vi "Filter and Data Scalingold1.vi"(0 "Offset Data":string[](array[string]), 5 "Slope Data":string[](array[string]), 7 "Filter Data":string[](array[string]), 9 "Vin":dbl[](array[numeric]), 11 "error in":errorcluster, 12 "Allow Zero?":string[](array[string])) -> (4 "Vout":string[](array[string]), 6 "Offset Data":string[](array[string]), 8 "ScaledOut":string[](array[string]), 10 "ScaledOut":dbl[](array[numeric]), 14 "Allow Zero?":string[](array[string]), 15 "error out":errorcluster)   [LabVIEW 2018]
uses:
  Counters.vi
  <vilib>/ptbypt/NI_PtbyPt.lvlib
panel:
  # "32-51= FM1 GPM Data Point 1-20"
  # "32-51= FM1 Data Point # 1-20"
  # "32-51 = FM1 K Factor 1-20"
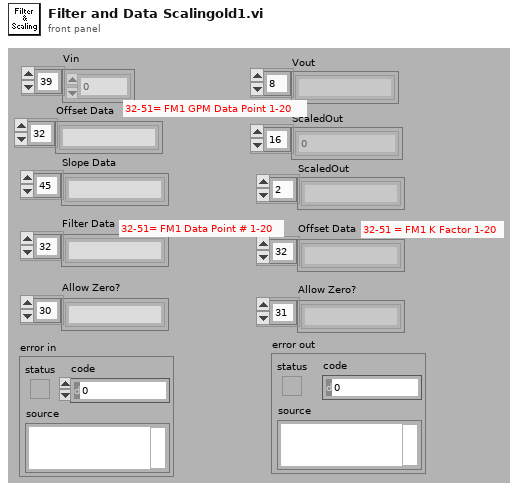
[diagram p1: front panel]
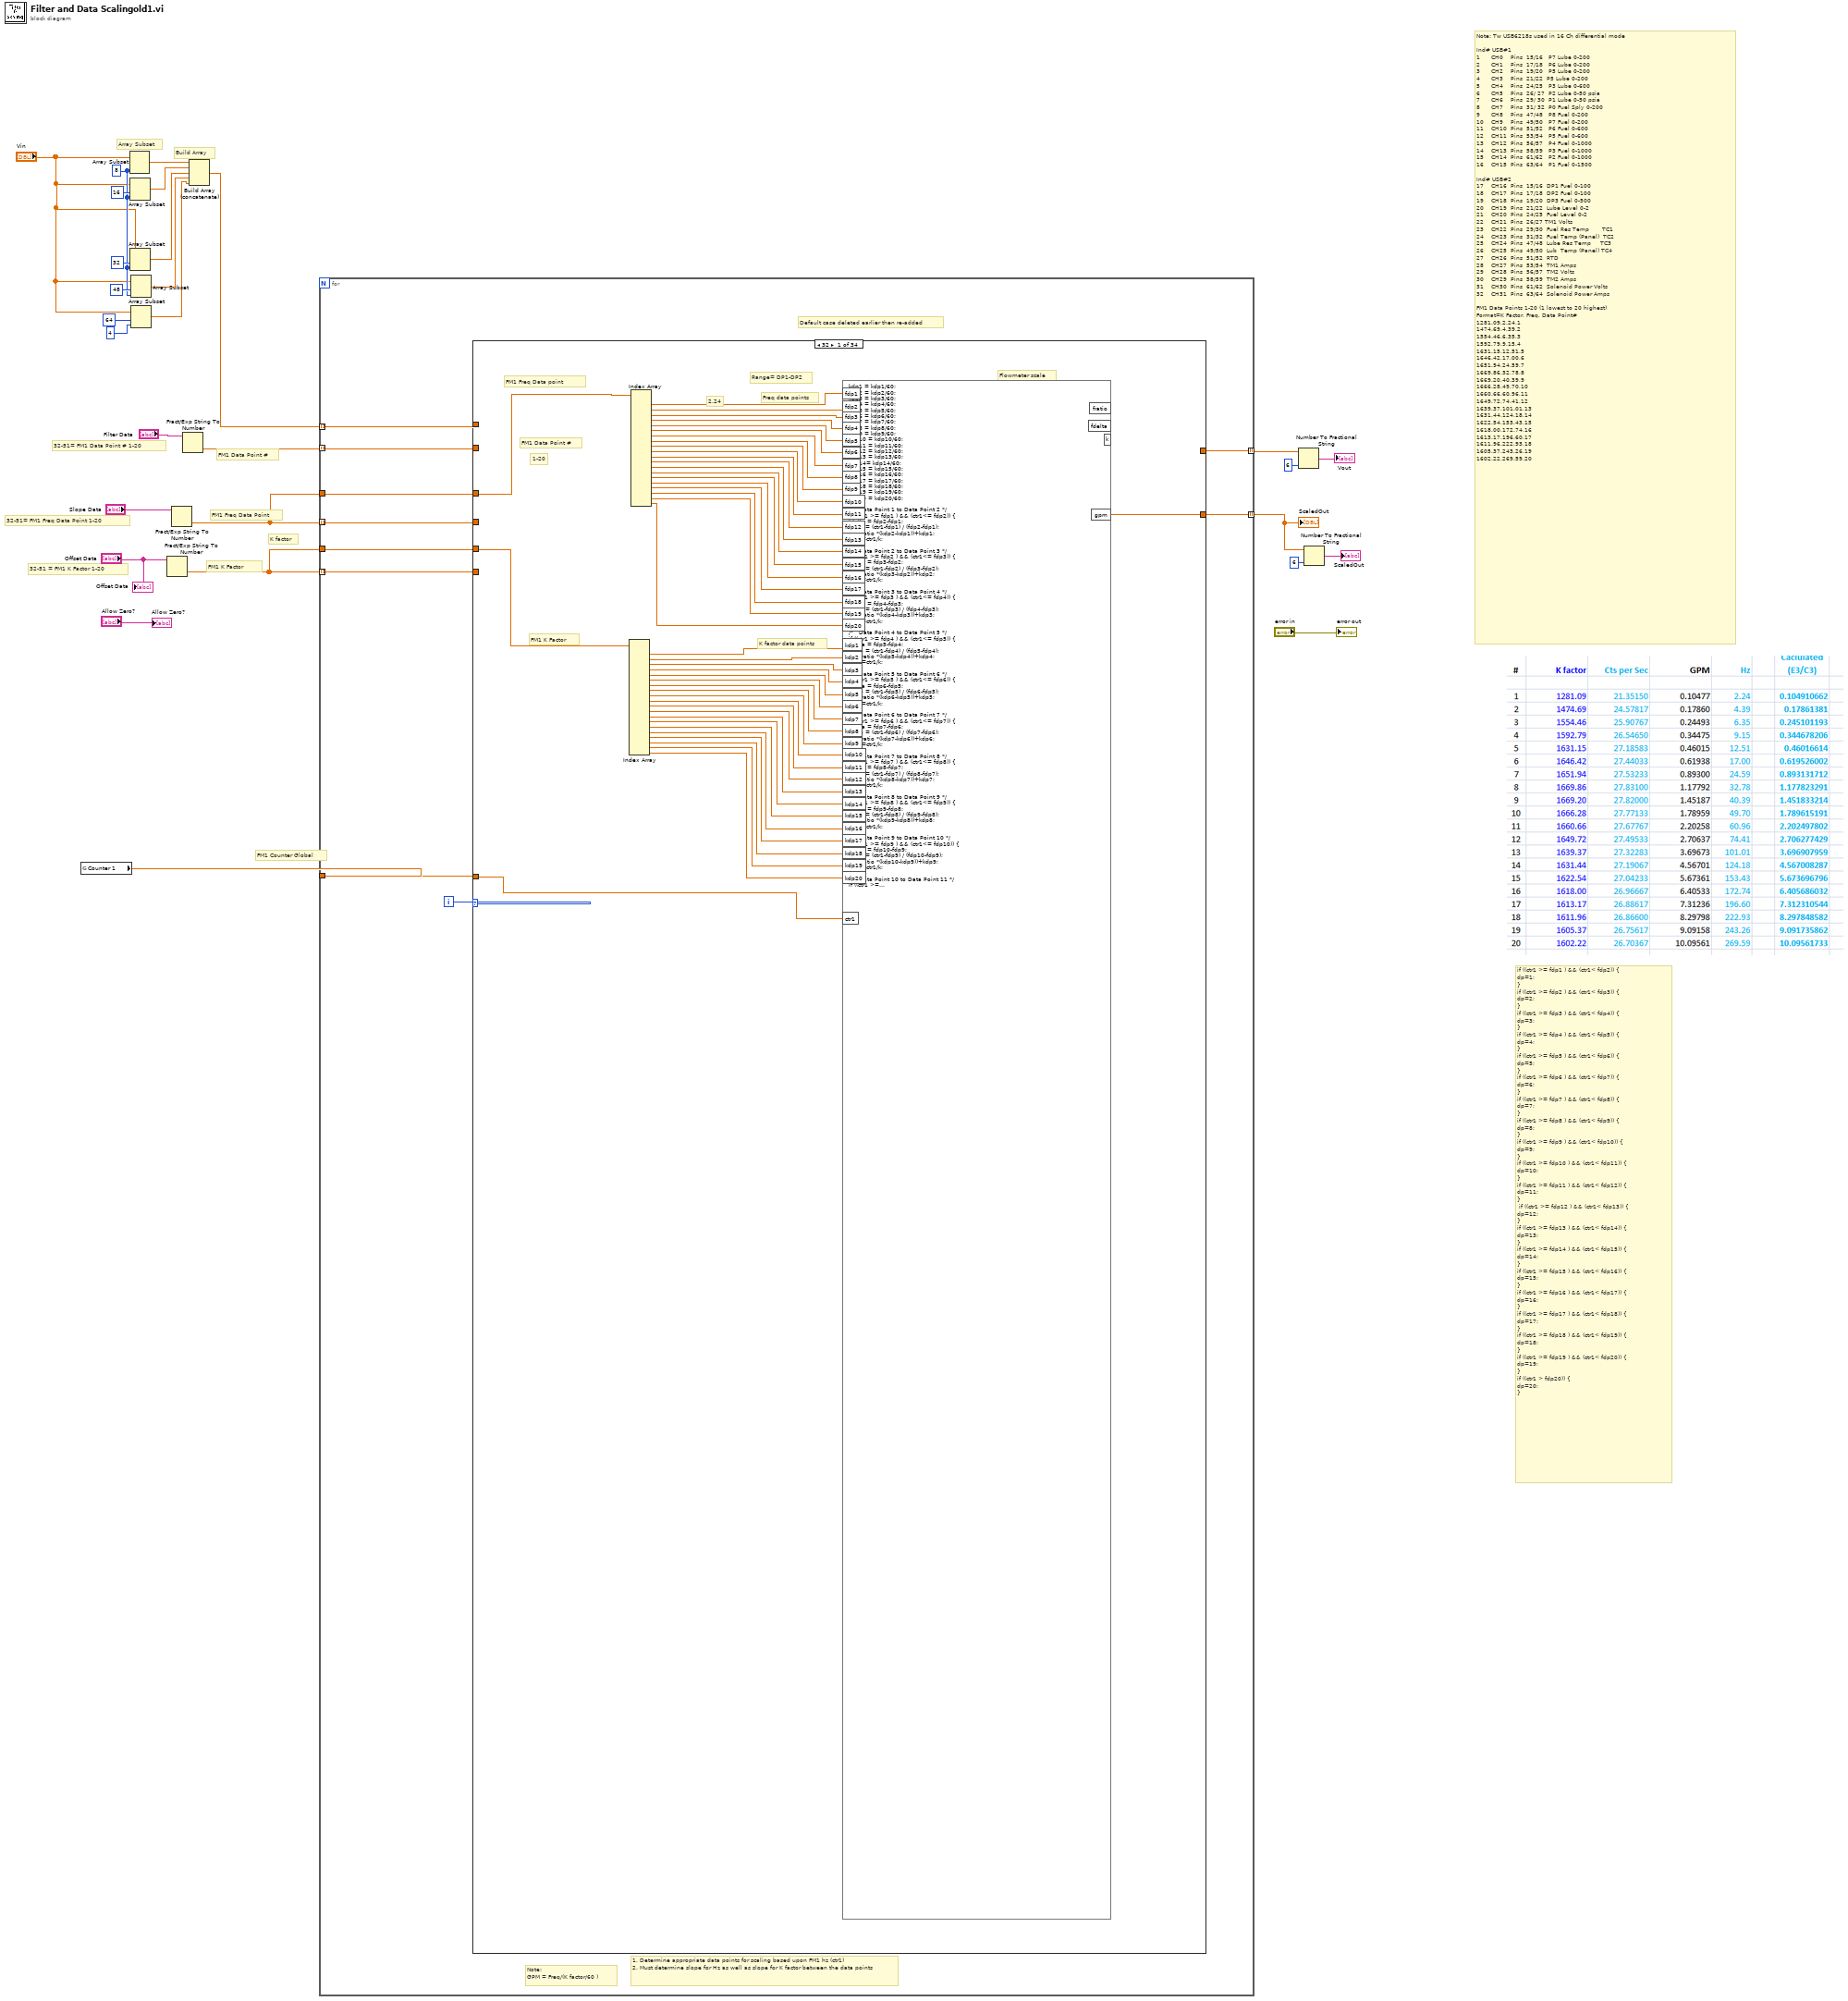
[diagram p0: block diagram]
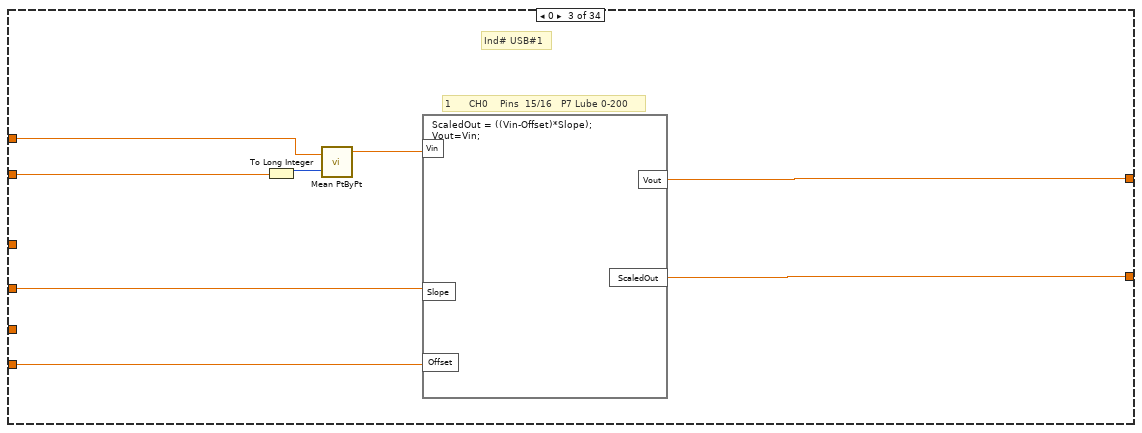
[diagram p3: hidden frame]
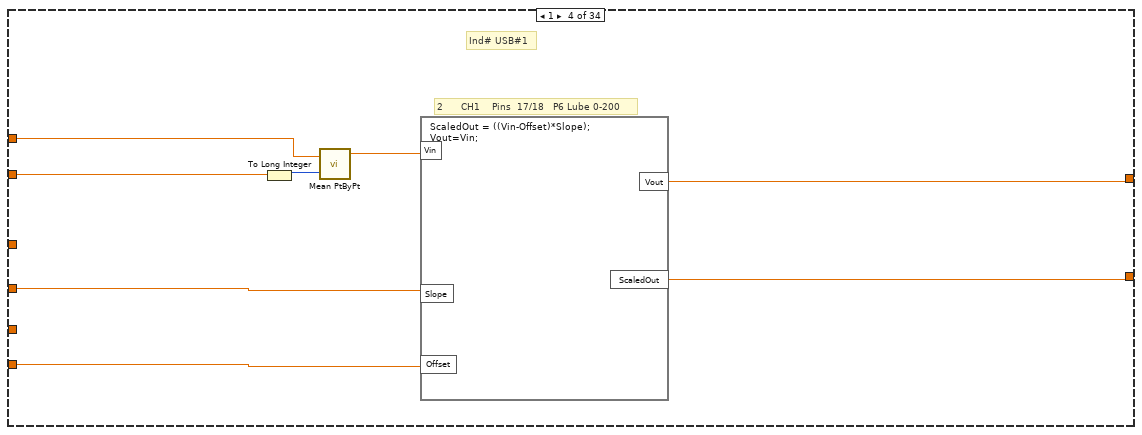
[diagram p4: hidden frame]
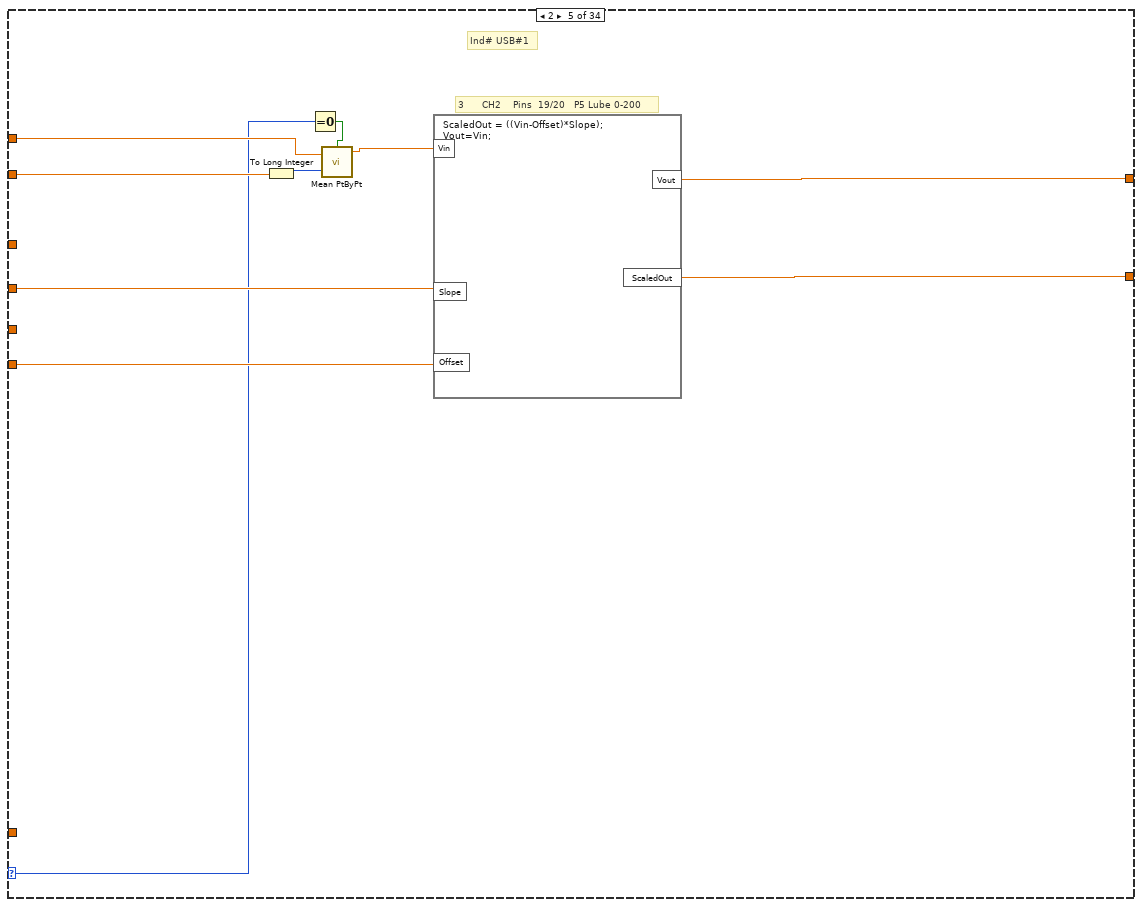
[diagram p5: hidden frame]
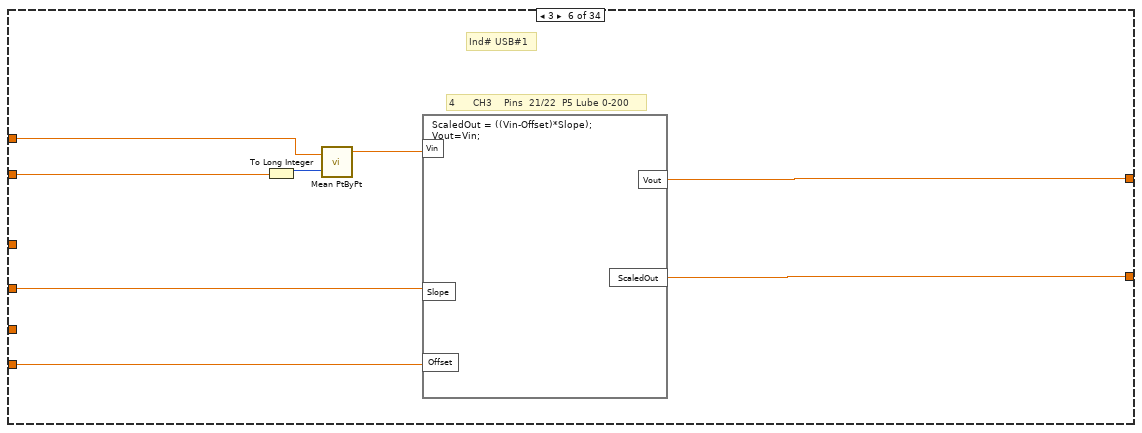
[diagram p6: hidden frame]
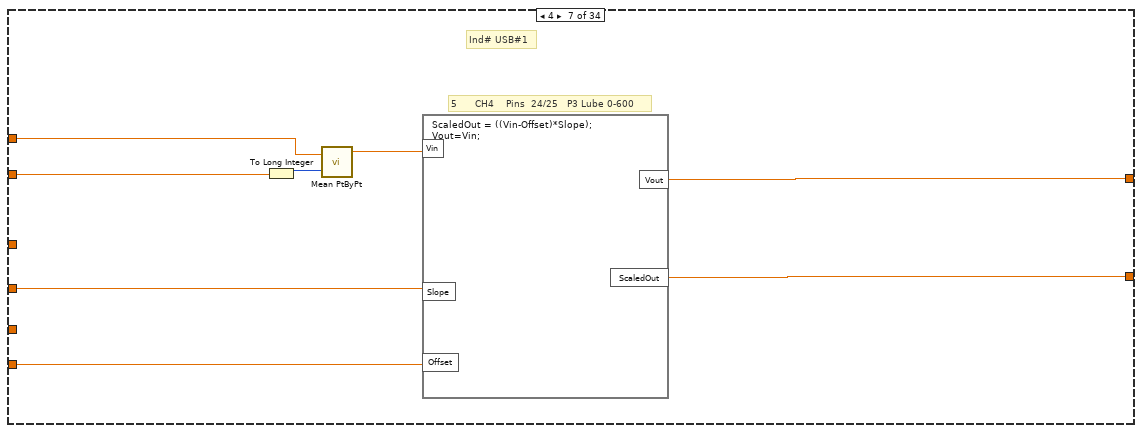
[diagram p7: hidden frame]
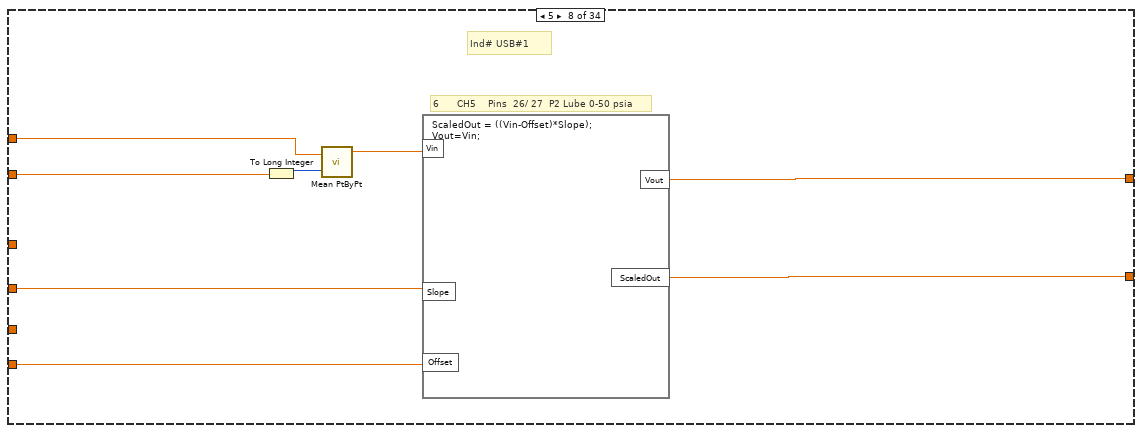
[diagram p8: hidden frame]
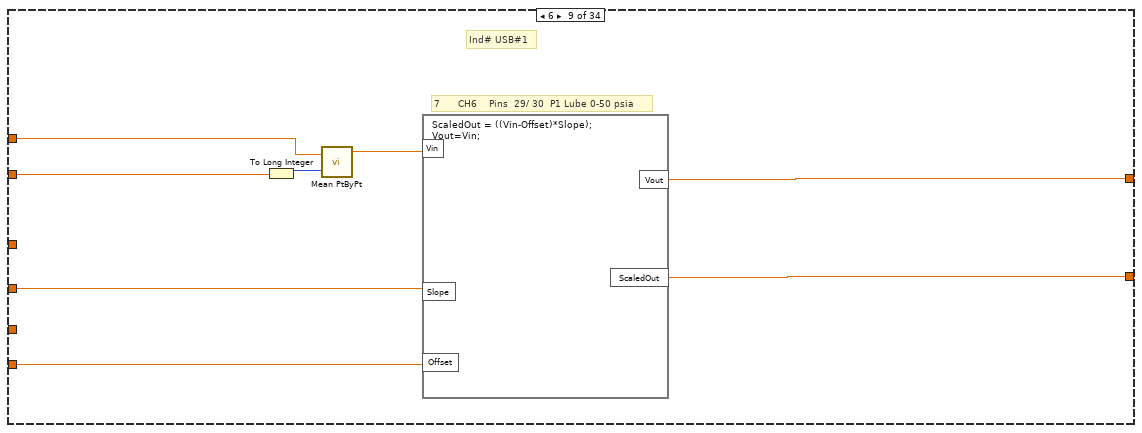
[diagram p9: hidden frame]
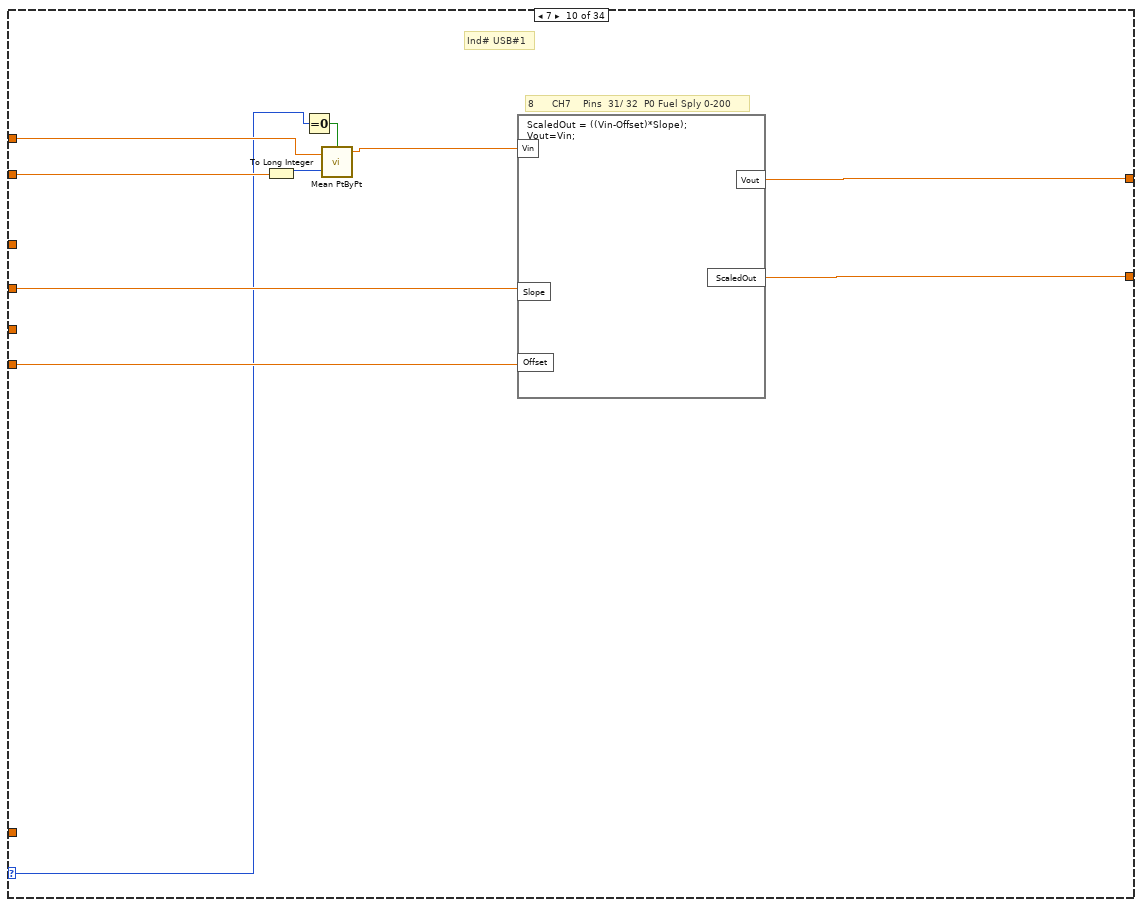
[diagram p10: hidden frame]
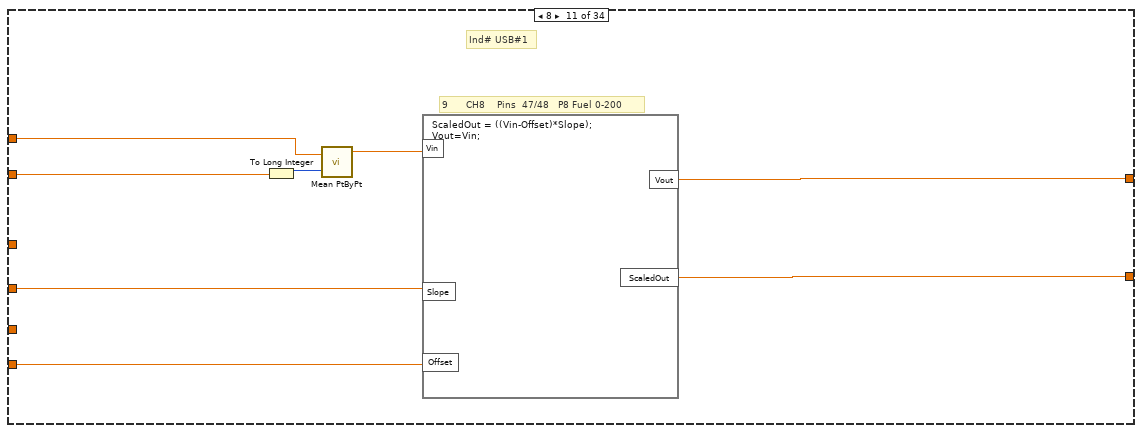
[diagram p11: hidden frame]
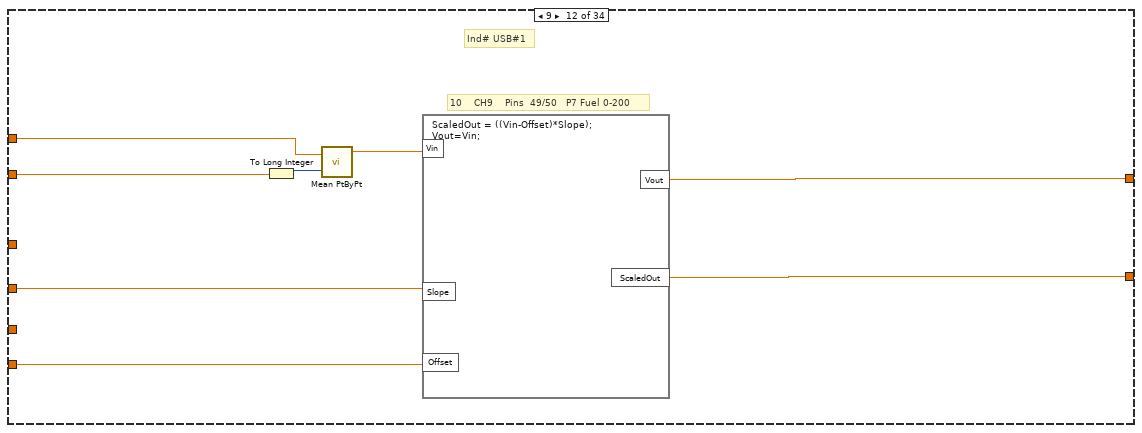
[diagram p12: hidden frame]
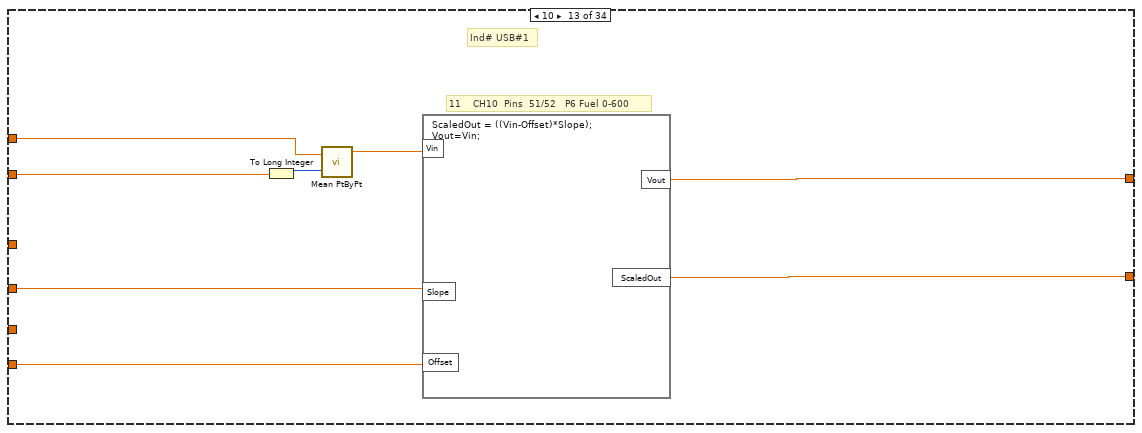
[diagram p13: hidden frame]
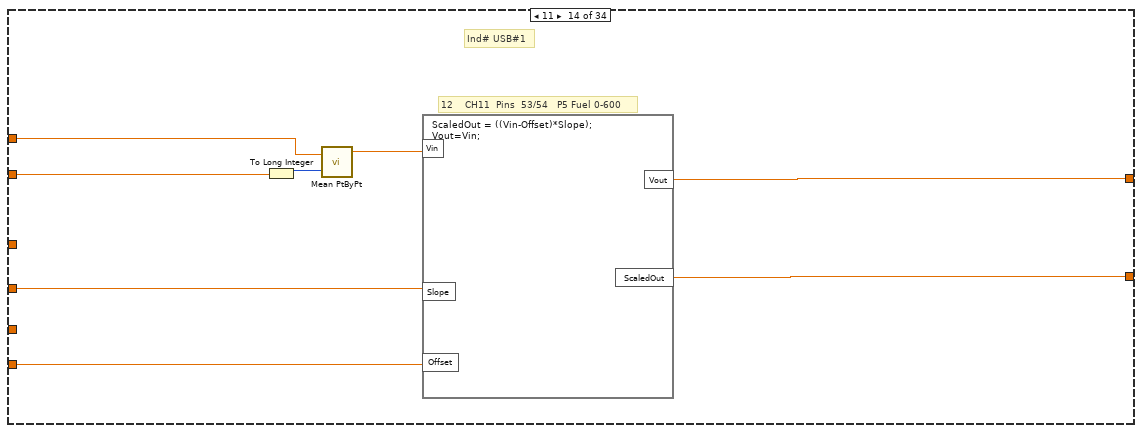
[diagram p14: hidden frame]
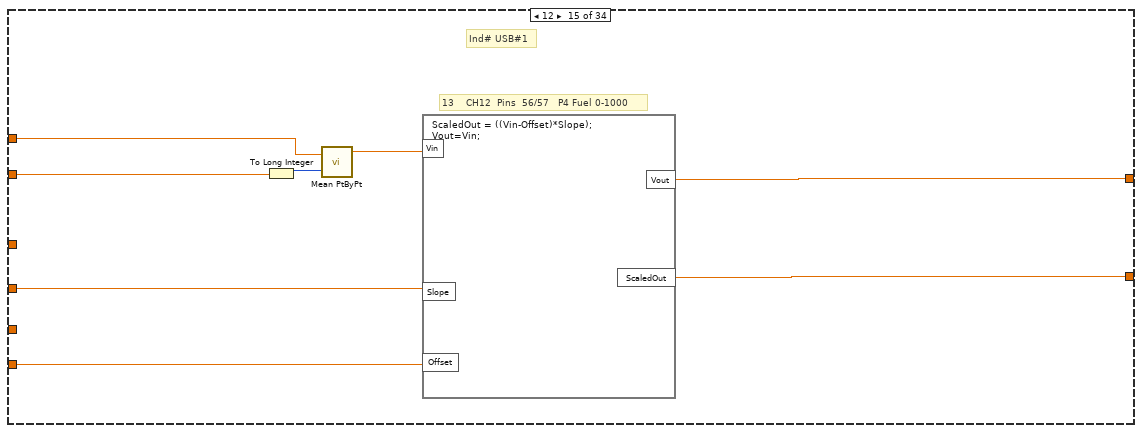
[diagram p15: hidden frame]
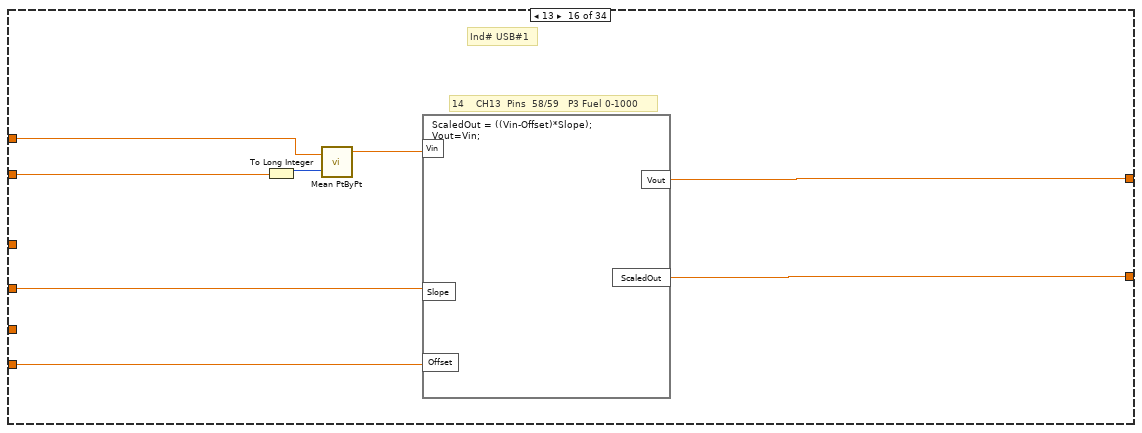
[diagram p16: hidden frame]
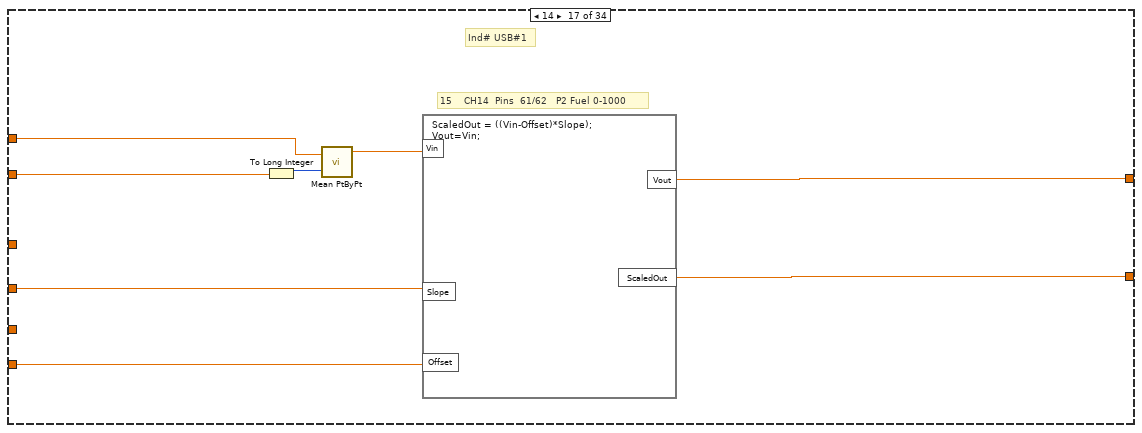
[diagram p17: hidden frame]
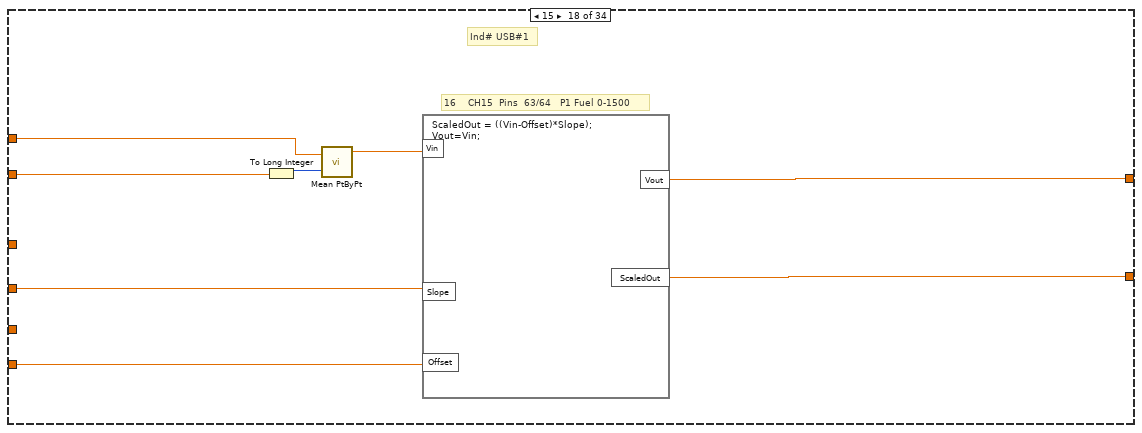
[diagram p18: hidden frame]
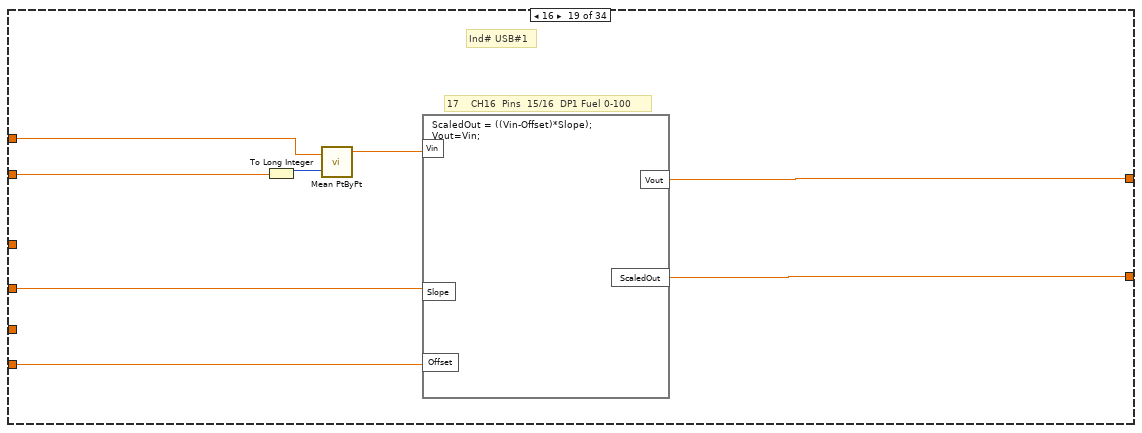
[diagram p19: hidden frame]
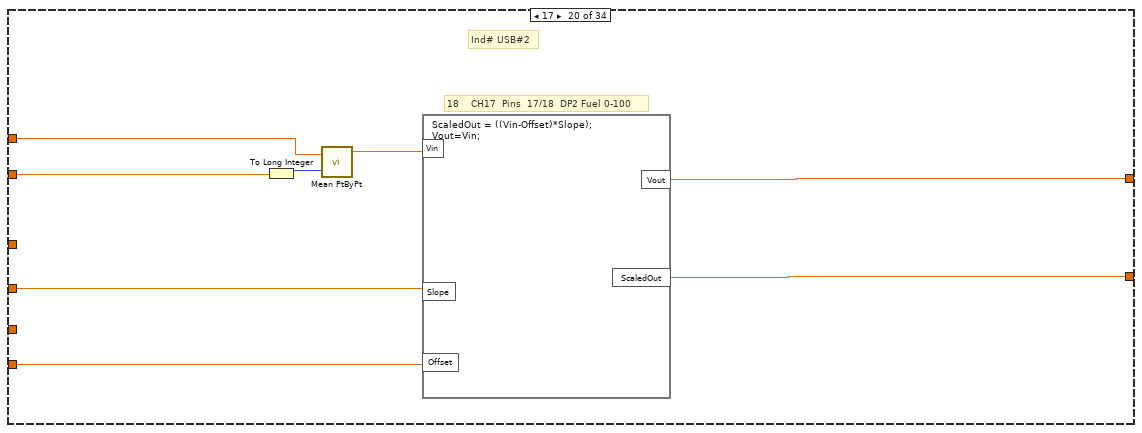
[diagram p20: hidden frame]
diagram:
  w11 = 8 ("length")
  # "if ((ctr1 >= fdp1 ) && (ctr1< fdp2)) {\ndp=1;\n}\nif ((ctr1 >= fdp2 ) && (ctr1< fdp3)) {\ndp=2;\n}\nif ((ctr1 >= fdp3 ) && (ctr1< fdp4)) {\ndp=3;\n}\nif ((ctr1 >= fdp4 ) && (ctr1< fdp5)) {\ndp=4;\n}\nif ((ctr1 >= fdp5 ) && (ctr1< fdp6)) {\ndp=5;\n}\nif ((ctr1 >= fdp6 ) && (ctr1< fdp7)) {\ndp=6;\n}\nif ((ctr1 >= fdp7 ) && (ctr1< fdp8)) {\ndp=7;\n}\nif ((ctr1 >= fdp8 ) && (ctr1< fdp9)) {\ndp=8;\n}\nif ((ctr1 >= fdp9 ) && (ctr1< fdp10)) {\ndp=9;\n}\nif ((ctr1 >= fdp10 ) && (ctr1< fdp11)) {\ndp=10;\n}\nif ((ctr1 >= fdp11 ) && (ctr1< fdp12)) {\ndp=11;\n}\n if ((ctr1 >= fdp12 ) && (ctr1< fdp13)) {\ndp=12;\n}\nif ((ctr1 >= fdp13 ) && (ctr1< fdp14)) {\ndp=13;\n}\nif ((ctr1 >= fdp14 ) && (ctr1< fdp15)) {\ndp=14;\n}\nif ((ctr1 >= fdp15 ) && (ctr1< fdp16)) {\ndp=15;\n}\nif ((ctr1 >= fdp16 ) && (ctr1< fdp17)) {\ndp=16;\n}\nif ((ctr1 >= fdp17 ) && (ctr1< fdp18)) {\ndp=17;\n}\nif ((ctr1 >= fdp18 ) && (ctr1< fdp19)) {\ndp=18;\n}\nif ((ctr1 >= fdp19 ) && (ctr1< fdp20)) {\ndp=19;\n}\nif ((ctr1 > fdp20)) {\ndp=20;\n}"
  # "Note: Tw USB6218s used in 16 Ch differential mode\n\nInd# USB#1\n1      CH0\t\t  Pins  15/16\t  P7 Lube 0-200\n2      CH1\t\t  Pins  17/18\t  P6 Lube 0-200\n3      CH2\t\t  Pins  19/20   P5 Lube 0-200\n4      CH3\t\t  Pins  21/22  P5 Lube 0-200\n5      CH4\t   Pins  24/25\t  P3 Lube 0-600\n6      CH5\t\t  Pins  26/\t27\t P2 Lube 0-50 psia\n7      CH6\t   Pins  29/\t30\t P1 Lube 0-50 psia\n8      CH7\t  \tPins  31/ 32\t P0 Fuel Sply 0-200  \n9      CH8\t  \tPins  47/48\t  P8 Fuel 0-200   \n10    CH9\t\t  Pins  49/50\t  P7 Fuel 0-200   \n11    CH10\t\tPins  51/52\t  P6 Fuel 0-600   \n12    CH11\t\tPins  53/54\t  P5 Fuel 0-600   \n13    CH12\t\tPins  56/57\t  P4 Fuel 0-1000 \n14    CH13\t\tPins  58/59\t  P3 Fuel 0-1000 \n15    CH14\t\tPins  61/62 \t P2 Fuel 0-1000  \n16    CH15\t\tPins  63/64 \t P1 Fuel 0-1500 \n\nInd# USB#2\n17    CH16\t\tPins  15/16\t DP1 Fuel 0-100 \n18    CH17\t\tPins  17/18\t DP2 Fuel 0-100\n19    CH18\t\tPins  19/20  DP3 Fuel 0-500 \n20    CH19\t Pins  21/22\t Lube Level 0-2 \n21    CH20\t\tPins  24/25\t Fuel Level 0-2 \n22    CH21\t\tPins  26/27\tTM1 Volts  \n23    CH22\t Pins  29/30  Fuel Res Temp       TC1\n24    CH23\t\tPins  31/32\t Fuel Temp (Panel)  TC2 \n25    CH24\t\tPins \t47/48\t Lube Res Temp     TC3 \n26    CH25\t\tPins  49/50\t Lub  Temp (Panel) TC4 \n27    CH26\t\tPins  51/52\t RTD \n28    CH27\t\tPins  53/54\t TM1 Amps \n29    CH28\t\tPins  56/57\t TM2 Volts\n30    CH29\t\tPins  58/59\t TM2 Amps \n31    CH30\t\tPins  61/62  Solenoid Power Volts \n32    CH31\t\tPins  63/64  Solenoid Power Amps\n\nFM1 Data Points 1-20 (1 lowest to 20 highest)\nFormat=K Factor, Freq, Data Point#\n1281.09,2.24,1\n1474.69,4.39,2\n1554.46,6.35,3\n1592.79,9.15,4\n1631.15,12.51,5\n1646.42,17.00,6\n1651.94,24.59,7\n1669.86,32.78,8\n1669.20,40.39,9\n1666.28,49.70,10\n1660.66,60.96,11\n1649.72,74.41,12\n1639.37,101.01,13\n1631.44,124.18,14\n1622.54,153.43,15\n1618.00,172.74,16\n1613.17,196.60,17\n1611.96,222.93,18\n1605.37,243.26,19\n1602.22,269.59,20"
  # "K factor"
  # "FM1 Freq Data Point"
  # "FM1 Counter Global"
  # "FM1 Data Point #"
  # "FM1 K Factor"
  # "32-51 = FM1 K Factor 1-20"
  # "32-51= FM1 Data Point # 1-20"
  # "32-51= FM1 Freq Data Point 1-20"
  # "Array Subset"
  # "Build Array"
  n1 = global read "Counters.vi" "Counter 1"() -> (w2:dbl)
  n2 = Array Subset(array="Vin", length=w11) -> (w16:dbl[])  [unwired: 1 in]
  n3 = Array Subset(array="Vin", index=16, length=w11) -> (w15:dbl[])
  n4 = Array Subset(array="Vin", index=32, length=w11) -> (w13:dbl[])
  n5 = Array Subset(array="Vin", index=48, length=w11) -> (w14:dbl[])
  n6 = Array Subset(array="Vin", index=64, length=4 ("index")) -> (w6:dbl[])
  n7 = Fract/Exp String To Number(string="Offset Data") -> (number=w3:dbl[])  [unwired: 4 out]
  n8 = Fract/Exp String To Number(string="Slope Data") -> (number=w4:dbl[])  [unwired: 4 out]
  n9 = Fract/Exp String To Number(string="Filter Data") -> (number=w1:dbl[])  [unwired: 4 out]
  n10 = Build Array (concatenate)(w16, w15, w13, w14, w6) -> (w5:dbl[])
  n11 = for {
    tunnel: w4 -> [w37] mode=indexing
    tunnel: w3 -> [w32] mode=indexing
    tunnel: w1 -> [w38] mode=indexing
    tunnel: [w35] -> w10 mode=indexing
    tunnel: [w36] -> w19 mode=indexing
    tunnel: w5 -> [w33] mode=indexing
    tunnel: w4 -> [w31]
    tunnel: w3 -> [w30]
    tunnel: w2 -> [w29]
    i -> [w34]
    # "Note:\nGPM = Freq/(K factor/60 )"
    # "1. Determine appropriate data points for scaling based upon FM1 hz (ctr1)\n2. Must determine slope for Hz as well as slope for K factor between the data points"
    # "Default case deleted earlier then re-added"
    n12 = case shown="32" w34 {
      selector: w34 -> [_ _ _ _ w102 _ _ _ _ w144 _ _ _ _ _ _ _ _ _ _ _ _ _ _ _ _ _ _ _ _ _ _ _ _]
      tunnel: w33 -> [_ _ w87 w93 w107 w113 w121 w129 w137 w149 w155 w163 w171 w179 w187 w195 w203 w211 w219 w227 w235 w243 w251 w259 w267 w275 w283 w291 w299 w307 w315 w323 w331 w339]
      tunnel: w38 -> [_ _ w88 w94 w108 w114 w122 w130 w138 w150 w156 w164 w172 w180 w188 w196 w204 w212 w220 w228 w236 w244 w252 w260 w268 w276 w284 w292 w300 w308 w316 w324 w332 w340]
      tunnel: w37 -> [_ _ w86 w96 w106 w112 w120 w128 w136 w148 w154 w162 w170 w178 w186 w194 w202 w210 w218 w226 w234 w242 w250 w258 w266 w274 w282 w290 w298 w306 w314 w322 w330 w338]
      tunnel: w32 -> [_ _ w85 w95 w105 w111 w119 w127 w135 w147 w153 w161 w169 w177 w185 w193 w201 w209 w217 w225 w233 w241 w249 w257 w265 w273 w281 w289 w297 w305 w313 w321 w329 w337]
      tunnel: [_ _ w83 w92 w103 w109 w117 w125 w133 w145 w151 w159 w167 w175 w183 w191 w199 w207 w215 w223 w231 w239 w247 w255 w263 w271 w279 w287 w295 w303 w311 w319 w327 w335] -> w36
      tunnel: [w79 _ w84 w91 w104 w110 w118 w126 w134 w146 w152 w160 w168 w176 w184 w192 w200 w208 w216 w224 w232 w240 w248 w256 w264 w272 w280 w288 w296 w304 w312 w320 w328 w336] -> w35
      tunnel: w31 -> [w81 _ _ _ _ _ _ _ _ _ _ _ _ _ _ _ _ _ _ _ _ _ _ _ _ _ _ _ _ _ _ _ _ _]
      tunnel: w30 -> [w80 _ _ _ _ _ _ _ _ _ _ _ _ _ _ _ _ _ _ _ _ _ _ _ _ _ _ _ _ _ _ _ _ _]
      tunnel: w29 -> [w82 _ _ _ _ _ _ _ _ _ _ _ _ _ _ _ _ _ _ _ _ _ _ _ _ _ _ _ _ _ _ _ _ _]
      frame 32 {
        # "2.24"
        # "Range= DP1-DP2"
        # "K factor data points"
        # "Freq data points"
        # "Flowmeter scale"
        # "1-20"
        # "FM1 Data Point #"
        # "FM1 K Factor"
        # "FM1 Freq Data point"
        n13 = Index Array(array=w80) -> (element #1=w58:dbl, element #2=w57:dbl, element #3=w56:dbl, element #4=w55:dbl, element #5=w54:dbl, element #6=w53:dbl, element #7=w52:dbl, element #8=w51:dbl, element #9=w50:dbl, element #10=w49:dbl, element #11=w48:dbl, element #12=w47:dbl, element #13=w46:dbl, element #14=w45:dbl, element #15=w44:dbl, element #16=w43:dbl, element #17=w42:dbl, element #18=w41:dbl, element #19=w40:dbl, element #20=w39:dbl)  [unwired: 20 in]
        n14 = Index Array(array=w81) -> (element #1=w78:dbl, element #2=w77:dbl, element #3=w76:dbl, element #4=w75:dbl, element #5=w74:dbl, element #6=w73:dbl, element #7=w72:dbl, element #8=w71:dbl, element #9=w70:dbl, element #10=w69:dbl, element #11=w68:dbl, element #12=w67:dbl, element #13=w66:dbl, element #14=w65:dbl, element #15=w64:dbl, element #16=w63:dbl, element #17=w62:dbl, element #18=w61:dbl, element #19=w60:dbl, element #20=w59:dbl)  [unwired: 20 in]
        n15 = formula code="kdp1 = kdp1/60;\nkdp2 = kdp2/60;\nkdp3 = kdp3/60;\nkdp4 = kdp4/60;\nkdp5 = kdp5/60;\nkdp6 = kdp6/60;\nkdp7 = kdp7/60;\nkdp8 = kdp8/60;\nkdp9 = kdp9/60;\nkdp10 = kdp10/60;\nkdp11 = kdp11/60;\nkdp12 = kdp12/60;\nkdp13 = kdp13/60;\nkdp14= kdp14/60;\nkdp15 = kdp15/60;\nkdp16 = kdp16/60;\nkdp17 = kdp17/60;\nkdp18 = kdp18/60;\nkdp19 = kdp19/60;\nkdp20 = kdp20/60;\n\n/*   Data Point 1 to Data Point 2 */\nif ((ctr1 >= fdp1 ) && (ctr1<= fdp2)) {\nfdelta = fdp2-fdp1;\nfratio = (ctr1-fdp1) / (fdp2-fdp1);\nk =(fratio *(kdp2-kdp1))+kdp1;\ngpm=ctr1/k;\n}\n/*   Data Point 2 to Data Point 3 */\nif ((ctr1 >= fdp2 ) && (ctr1<= fdp3)) {\nfdelta = fdp3-fdp2;\nfratio = (ctr1-fdp2) / (fdp3-fdp2);\nk =(fratio *(kdp3-kdp2))+kdp2;\ngpm=ctr1/k;\n}\n/*   Data Point 3 to Data Point 4 */\nif ((ctr1 >= fdp3 ) && (ctr1<= fdp4)) {\nfdelta = fdp4-fdp3;\nfratio = (ctr1-fdp3) / (fdp4-fdp3);\nk =(fratio *(kdp4-kdp3))+kdp3;\ngpm=ctr1/k;\n}\n/*   Data Point 4 to Data Point 5 */\nif ((ctr1 >= fdp4 ) && (ctr1<= fdp5)) {\nfdelta = fdp5-fdp4;\nfratio = (ctr1-fdp4) / (fdp5-fdp4);\nk =(fratio *(kdp5-kdp4))+kdp4;\ngpm=ctr1/k;\n}\n/*   Data Point 5 to Data Point 6 */\nif ((ctr1 >= fdp5 ) && (ctr1<= fdp6)) {\nfdelta = fdp6-fdp5;\nfratio = (ctr1-fdp5) / (fdp6-fdp5);\nk =(fratio *(kdp6-kdp5))+kdp5;\ngpm=ctr1/k;\n}\n/*   Data Point 6 to Data Point 7 */\nif ((ctr1 >= fdp6 ) && (ctr1<= fdp7)) {\nfdelta = fdp7-fdp6;\nfratio = (ctr1-fdp6) / (fdp7-fdp6);\nk =(fratio *(kdp7-kdp6))+kdp6;\ngpm=ctr1/k;\n}\n/*   Data Point 7 to Data Point 8 */\nif ((ctr1 >= fdp7 ) && (ctr1<= fdp8)) {\nfdelta = fdp8-fdp7;\nfratio = (ctr1-fdp7) / (fdp8-fdp7);\nk =(fratio *(kdp8-kdp7))+kdp7;\ngpm=ctr1/k;\n}\n/*   Data Point 8 to Data Point 9 */\nif ((ctr1 >= fdp8 ) && (ctr1<= fdp9)) {\nfdelta = fdp9-fdp8;\nfratio = (ctr1-fdp8) / (fdp9-fdp8);\nk =(fratio *(kdp9-kdp8))+kdp8;\ngpm=ctr1/k;\n}\n/*   Data Point 9 to Data Point 10 */\nif ((ctr1 >= fdp9 ) && (ctr1<= fdp10)) {\nfdelta = fdp10-fdp9;\nfratio = (ctr1-fdp9) / (fdp10-fdp9);\nk =(fratio *(kdp10-kdp9))+kdp9;\ngpm=ctr1/k;\n}\n/*   Data Point 10 to Data Point 11 */\nif ((ctr1 >= fdp10 ) && (ctr1<= fdp11)) {\nfdelta = fdp11-fdp10;\nfratio = (ctr1-fdp10) / (fdp11-fdp10);\nk =(fratio *(kdp11-kdp10))+kdp10;\ngpm=ctr1/k;\n}\n/*   Data Point 11 to Data Point 12 */\nif ((ctr1 >= fdp11 ) && (ctr1<= fdp12)) {\nfdelta = fdp12-fdp11;\nfratio = (ctr1-fdp11) / (fdp12-fdp11);\nk =(fratio *(kdp12-kdp11))+kdp11;\ngpm=ctr1/k;\n}\n/*   Data Point 12 to Data Point 13 */\nif ((ctr1 >= fdp12) && (ctr1<= fdp13)) {\nfdelta = fdp13-fdp12;\nfratio = (ctr1-fdp12) / (fdp13-fdp12);\nk =(fratio *(kdp13-kdp12))+kdp12;\ngpm=ctr1/k;\n}\n/*   Data Point 13 to Data Point 14 */\nif ((ctr1 >= fdp13 ) && (ctr1<= fdp14)) {\nfdelta = fdp14-fdp13;\nfratio = (ctr1-fdp13) / (fdp14-fdp13);\nk =(fratio *(kdp14-kdp13))+kdp13;\ngpm=ctr1/k;\n}\nif ((ctr1 >= fdp14 ) && (ctr1<= fdp15)) {\nfdelta = fdp15-fdp14;\nfratio = (ctr1-fdp14) / (fdp15-fdp14);\nk =(fratio *(kdp15-kdp14))+kdp14;\ngpm=ctr1/k;\n}\n/*   Data Point 15 to Data Point 16 */\nif ((ctr1 >= fdp15 ) && (ctr1<= fdp16)) {\nfdelta = fdp16-fdp15;\nfratio = (ctr1-fdp15) / (fdp16-fdp15);\nk =(fratio *(kdp16-kdp15))+kdp15;\ngpm=ctr1/k;\n}\n/*   Data Point 16 to Data Point 17 */\nif ((ctr1 >= fdp16 ) && (ctr1<= fdp17)) {\nfdelta = fdp17-fdp16;\nfratio = (ctr1-fdp16) / (fdp17-fdp16);\nk =(fratio *(kdp17-kdp16))+kdp16;\ngpm=ctr1/k;\n}\n/*   Data Point 17 to Data Point 18 */\nif ((ctr1 >= fdp17 ) && (ctr1<= fdp18)) {\nfdelta = fdp18-fdp17;\nfratio = (ctr1-fdp17) / (fdp18-fdp17);\nk =(fratio *(kdp18-kdp17))+kdp17;\ngpm=ctr1/k;\n}\n/*   Data Point 18 to Data Point 19 */\nif ((ctr1 >= fdp18 ) && (ctr1<= fdp19)) {\nfdelta = fdp19-fdp18;\nfratio = (ctr1-fdp18) / (fdp19-fdp18);\nk =(fratio *(kdp19-kdp18))+kdp18;\ngpm=ctr1/k;\n}\n/*   Data Point 19 to Data Point 20 */\nif ((ctr1 >= fdp19 ) && (ctr1<= fdp20)) {\nfdelta = fdp20-fdp19;\nfratio = (ctr1-fdp19) / (fdp20-fdp19);\nk =(fratio *(kdp20-kdp19))+kdp19;\ngpm=ctr1/k;\n}\n\nif (ctr1 < fdp1) {  /*  Handles frequency < lowest on table */ \ngpm =0;\n}"("fdp1"=w78, "fdp2"=w77, "kdp1"=w58, "ctr1"=w82, "kdp2"=w57, "fdp3"=w76, "fdp4"=w75, "fdp5"=w74, "fdp6"=w73, "fdp7"=w72, "fdp8"=w71, "fdp9"=w70, "fdp10"=w69, "fdp11"=w68, "fdp12"=w67, "fdp13"=w66, "fdp14"=w65, "fdp15"=w64, "fdp16"=w63, "fdp17"=w62, "fdp18"=w61, "fdp19"=w60, "fdp20"=w59, "kdp3"=w56, "kdp4"=w55, "kdp5"=w54, "kdp6"=w53, "kdp7"=w52, "kdp8"=w51, "kdp9"=w50, "kdp10"=w49, "kdp11"=w48, "kdp12"=w47, "kdp13"=w46, "kdp14"=w45, "kdp15"=w44, "kdp16"=w43, "kdp17"=w42, "kdp18"=w41, "kdp19"=w40, "kdp20"=w39) -> ("gpm"=w79:dbl)  [unwired: 3 out]
      }
      frame 33, Default {
      }
      frame 0 {
        # "Ind# USB#1"
        # "1      CH0\t\t  Pins  15/16\t  P7 Lube 0-200"
        n16 = To Long Integer(number=w88) -> (32bit integer=w90:i32)
        n17 = call <vilib>:"Mean PtByPt.vi"("x"=w87, "sample length"=w90) -> ("mean"=w89:dbl)  [unwired: 1 in, 2 out]
        n18 = formula code="ScaledOut = ((Vin-Offset)*Slope);\nVout=Vin;"("Vin"=w89, "Slope"=w86, "Offset"=w85) -> ("ScaledOut"=w84:dbl, "Vout"=w83:dbl)
      }
      frame 1 {
        # "Ind# USB#1"
        # "2      CH1\t\t  Pins  17/18\t  P6 Lube 0-200"
        n19 = To Long Integer(number=w94) -> (32bit integer=w98:i32)
        n20 = call <vilib>:"Mean PtByPt.vi"("x"=w93, "sample length"=w98) -> ("mean"=w97:dbl)  [unwired: 1 in, 2 out]
        n21 = formula code="ScaledOut = ((Vin-Offset)*Slope);\nVout=Vin;"("Vin"=w97, "Slope"=w96, "Offset"=w95) -> ("ScaledOut"=w91:dbl, "Vout"=w92:dbl)
      }
      frame 2 {
        # "Ind# USB#1"
        # "3      CH2\t\t  Pins  19/20   P5 Lube 0-200"
        n22 = To Long Integer(number=w108) -> (32bit integer=w101:i32)
        n23 = Equal To 0?(x=w102) -> (x = 0?=w100:bool)
        n24 = call <vilib>:"Mean PtByPt.vi"("x"=w107, "sample length"=w101, "initialize"=w100) -> ("mean"=w99:dbl)  [unwired: 2 out]
        n25 = formula code="ScaledOut = ((Vin-Offset)*Slope);\nVout=Vin;"("Vin"=w99, "Slope"=w106, "Offset"=w105) -> ("ScaledOut"=w104:dbl, "Vout"=w103:dbl)
      }
      frame 3 {
        # "Ind# USB#1"
        # "4      CH3\t\t  Pins  21/22  P5 Lube 0-200"
        n26 = To Long Integer(number=w114) -> (32bit integer=w116:i32)
        n27 = call <vilib>:"Mean PtByPt.vi"("x"=w113, "sample length"=w116) -> ("mean"=w115:dbl)  [unwired: 1 in, 2 out]
        n28 = formula code="ScaledOut = ((Vin-Offset)*Slope);\nVout=Vin;"("Vin"=w115, "Slope"=w112, "Offset"=w111) -> ("ScaledOut"=w110:dbl, "Vout"=w109:dbl)
      }
      frame 4 {
        # "Ind# USB#1"
        # "5      CH4\t   Pins  24/25\t  P3 Lube 0-600"
        n29 = To Long Integer(number=w122) -> (32bit integer=w124:i32)
        n30 = call <vilib>:"Mean PtByPt.vi"("x"=w121, "sample length"=w124) -> ("mean"=w123:dbl)  [unwired: 1 in, 2 out]
        n31 = formula code="ScaledOut = ((Vin-Offset)*Slope);\nVout=Vin;"("Vin"=w123, "Slope"=w120, "Offset"=w119) -> ("ScaledOut"=w118:dbl, "Vout"=w117:dbl)
      }
      frame 5 {
        # "6      CH5\t\t  Pins  26/\t27\t P2 Lube 0-50 psia"
        # "Ind# USB#1"
        n32 = To Long Integer(number=w130) -> (32bit integer=w132:i32)
        n33 = call <vilib>:"Mean PtByPt.vi"("x"=w129, "sample length"=w132) -> ("mean"=w131:dbl)  [unwired: 1 in, 2 out]
        n34 = formula code="ScaledOut = ((Vin-Offset)*Slope);\nVout=Vin;"("Vin"=w131, "Slope"=w128, "Offset"=w127) -> ("ScaledOut"=w126:dbl, "Vout"=w125:dbl)
      }
      frame 6 {
        # "7      CH6\t   Pins  29/\t30\t P1 Lube 0-50 psia"
        # "Ind# USB#1"
        n35 = To Long Integer(number=w138) -> (32bit integer=w140:i32)
        n36 = call <vilib>:"Mean PtByPt.vi"("x"=w137, "sample length"=w140) -> ("mean"=w139:dbl)  [unwired: 1 in, 2 out]
        n37 = formula code="ScaledOut = ((Vin-Offset)*Slope);\nVout=Vin;"("Vin"=w139, "Slope"=w136, "Offset"=w135) -> ("ScaledOut"=w134:dbl, "Vout"=w133:dbl)
      }
      frame 7 {
        # "8      CH7\t  \tPins  31/ 32\t P0 Fuel Sply 0-200"
        # "Ind# USB#1"
        n38 = To Long Integer(number=w150) -> (32bit integer=w142:i32)
        n39 = Equal To 0?(x=w144) -> (x = 0?=w143:bool)
        n40 = call <vilib>:"Mean PtByPt.vi"("x"=w149, "sample length"=w142, "initialize"=w143) -> ("mean"=w141:dbl)  [unwired: 2 out]
        n41 = formula code="ScaledOut = ((Vin-Offset)*Slope);\nVout=Vin;"("Vin"=w141, "Slope"=w148, "Offset"=w147) -> ("ScaledOut"=w146:dbl, "Vout"=w145:dbl)
      }
      frame 8 {
        # "9      CH8\t  \tPins  47/48\t  P8 Fuel 0-200"
        # "Ind# USB#1"
        n42 = To Long Integer(number=w156) -> (32bit integer=w158:i32)
        n43 = call <vilib>:"Mean PtByPt.vi"("x"=w155, "sample length"=w158) -> ("mean"=w157:dbl)  [unwired: 1 in, 2 out]
        n44 = formula code="ScaledOut = ((Vin-Offset)*Slope);\nVout=Vin;"("Vin"=w157, "Slope"=w154, "Offset"=w153) -> ("ScaledOut"=w152:dbl, "Vout"=w151:dbl)
      }
      frame 9 {
        # "10    CH9\t\t  Pins  49/50\t  P7 Fuel 0-200"
        # "Ind# USB#1"
        n45 = To Long Integer(number=w164) -> (32bit integer=w166:i32)
        n46 = call <vilib>:"Mean PtByPt.vi"("x"=w163, "sample length"=w166) -> ("mean"=w165:dbl)  [unwired: 1 in, 2 out]
        n47 = formula code="ScaledOut = ((Vin-Offset)*Slope);\nVout=Vin;"("Vin"=w165, "Slope"=w162, "Offset"=w161) -> ("ScaledOut"=w160:dbl, "Vout"=w159:dbl)
      }
      frame 10 {
        # "11    CH10\t\tPins  51/52\t  P6 Fuel 0-600"
        # "Ind# USB#1"
        n48 = To Long Integer(number=w172) -> (32bit integer=w174:i32)
        n49 = call <vilib>:"Mean PtByPt.vi"("x"=w171, "sample length"=w174) -> ("mean"=w173:dbl)  [unwired: 1 in, 2 out]
        n50 = formula code="ScaledOut = ((Vin-Offset)*Slope);\nVout=Vin;"("Vin"=w173, "Slope"=w170, "Offset"=w169) -> ("ScaledOut"=w168:dbl, "Vout"=w167:dbl)
      }
      frame 11 {
        # "12    CH11\t\tPins  53/54\t  P5 Fuel 0-600"
        # "Ind# USB#1"
        n51 = To Long Integer(number=w180) -> (32bit integer=w182:i32)
        n52 = call <vilib>:"Mean PtByPt.vi"("x"=w179, "sample length"=w182) -> ("mean"=w181:dbl)  [unwired: 1 in, 2 out]
        n53 = formula code="ScaledOut = ((Vin-Offset)*Slope);\nVout=Vin;"("Vin"=w181, "Slope"=w178, "Offset"=w177) -> ("ScaledOut"=w176:dbl, "Vout"=w175:dbl)
      }
      frame 12 {
        # "13    CH12\t\tPins  56/57\t  P4 Fuel 0-1000"
        # "Ind# USB#1"
        n54 = To Long Integer(number=w188) -> (32bit integer=w190:i32)
        n55 = call <vilib>:"Mean PtByPt.vi"("x"=w187, "sample length"=w190) -> ("mean"=w189:dbl)  [unwired: 1 in, 2 out]
        n56 = formula code="ScaledOut = ((Vin-Offset)*Slope);\nVout=Vin;"("Vin"=w189, "Slope"=w186, "Offset"=w185) -> ("ScaledOut"=w184:dbl, "Vout"=w183:dbl)
      }
      frame 13 {
        # "14    CH13\t\tPins  58/59\t  P3 Fuel 0-1000"
        # "Ind# USB#1"
        n57 = To Long Integer(number=w196) -> (32bit integer=w198:i32)
        n58 = call <vilib>:"Mean PtByPt.vi"("x"=w195, "sample length"=w198) -> ("mean"=w197:dbl)  [unwired: 1 in, 2 out]
        n59 = formula code="ScaledOut = ((Vin-Offset)*Slope);\nVout=Vin;"("Vin"=w197, "Slope"=w194, "Offset"=w193) -> ("ScaledOut"=w192:dbl, "Vout"=w191:dbl)
      }
      frame 14 {
        # "15    CH14\t\tPins  61/62 \t P2 Fuel 0-1000"
        # "Ind# USB#1"
        n60 = To Long Integer(number=w204) -> (32bit integer=w206:i32)
        n61 = call <vilib>:"Mean PtByPt.vi"("x"=w203, "sample length"=w206) -> ("mean"=w205:dbl)  [unwired: 1 in, 2 out]
        n62 = formula code="ScaledOut = ((Vin-Offset)*Slope);\nVout=Vin;"("Vin"=w205, "Slope"=w202, "Offset"=w201) -> ("ScaledOut"=w200:dbl, "Vout"=w199:dbl)
      }
      frame 15 {
        # "16    CH15\t\tPins  63/64 \t P1 Fuel 0-1500"
        # "Ind# USB#1"
        n63 = To Long Integer(number=w212) -> (32bit integer=w214:i32)
        n64 = call <vilib>:"Mean PtByPt.vi"("x"=w211, "sample length"=w214) -> ("mean"=w213:dbl)  [unwired: 1 in, 2 out]
        n65 = formula code="ScaledOut = ((Vin-Offset)*Slope);\nVout=Vin;"("Vin"=w213, "Slope"=w210, "Offset"=w209) -> ("ScaledOut"=w208:dbl, "Vout"=w207:dbl)
      }
      frame 16 {
        # "17    CH16\t\tPins  15/16\t DP1 Fuel 0-100"
        # "Ind# USB#1"
        n66 = To Long Integer(number=w220) -> (32bit integer=w222:i32)
        n67 = call <vilib>:"Mean PtByPt.vi"("x"=w219, "sample length"=w222) -> ("mean"=w221:dbl)  [unwired: 1 in, 2 out]
        n68 = formula code="ScaledOut = ((Vin-Offset)*Slope);\nVout=Vin;"("Vin"=w221, "Slope"=w218, "Offset"=w217) -> ("ScaledOut"=w216:dbl, "Vout"=w215:dbl)
      }
      frame 17 {
        # "18    CH17\t\tPins  17/18\t DP2 Fuel 0-100"
        # "Ind# USB#2"
        n69 = To Long Integer(number=w228) -> (32bit integer=w230:i32)
        n70 = call <vilib>:"Mean PtByPt.vi"("x"=w227, "sample length"=w230) -> ("mean"=w229:dbl)  [unwired: 1 in, 2 out]
        n71 = formula code="ScaledOut = ((Vin-Offset)*Slope);\nVout=Vin;"("Vin"=w229, "Slope"=w226, "Offset"=w225) -> ("ScaledOut"=w224:dbl, "Vout"=w223:dbl)
      }
      frame 18 {
        # "19    CH18\t\tPins  19/20  DP3 Fuel 0-500"
        # "Ind# USB#2"
        n72 = To Long Integer(number=w236) -> (32bit integer=w238:i32)
        n73 = call <vilib>:"Mean PtByPt.vi"("x"=w235, "sample length"=w238) -> ("mean"=w237:dbl)  [unwired: 1 in, 2 out]
        n74 = formula code="ScaledOut = ((Vin-Offset)*Slope);\nVout=Vin;"("Vin"=w237, "Slope"=w234, "Offset"=w233) -> ("ScaledOut"=w232:dbl, "Vout"=w231:dbl)
      }
      frame 19 {
        # "20    CH19\t Pins  21/22\t Lube Level 0-2"
        # "Ind# USB#2"
        n75 = To Long Integer(number=w244) -> (32bit integer=w246:i32)
        n76 = call <vilib>:"Mean PtByPt.vi"("x"=w243, "sample length"=w246) -> ("mean"=w245:dbl)  [unwired: 1 in, 2 out]
        n77 = formula code="ScaledOut = ((Vin-Offset)*Slope);\nVout=Vin;"("Vin"=w245, "Slope"=w242, "Offset"=w241) -> ("ScaledOut"=w240:dbl, "Vout"=w239:dbl)
      }
      frame 20 {
        # "21    CH20\t\tPins  24/25\t Fuel Level 0-2"
        # "Ind# USB#2"
        n78 = To Long Integer(number=w252) -> (32bit integer=w254:i32)
        n79 = call <vilib>:"Mean PtByPt.vi"("x"=w251, "sample length"=w254) -> ("mean"=w253:dbl)  [unwired: 1 in, 2 out]
        n80 = formula code="ScaledOut = ((Vin-Offset)*Slope);\nVout=Vin;"("Vin"=w253, "Slope"=w250, "Offset"=w249) -> ("ScaledOut"=w248:dbl, "Vout"=w247:dbl)
      }
      frame 21 {
        # "22    CH21\t\tPins  26/27\tTM1 Volts"
        # "Ind# USB#2"
        n81 = To Long Integer(number=w260) -> (32bit integer=w262:i32)
        n82 = call <vilib>:"Mean PtByPt.vi"("x"=w259, "sample length"=w262) -> ("mean"=w261:dbl)  [unwired: 1 in, 2 out]
        n83 = formula code="ScaledOut = ((Vin-Offset)*Slope);\nVout=Vin;"("Vin"=w261, "Slope"=w258, "Offset"=w257) -> ("ScaledOut"=w256:dbl, "Vout"=w255:dbl)
      }
      frame 22 {
        # "23    CH22\t Pins  29/30  Fuel Res Temp       TC1"
        # "Ind# USB#2"
        n84 = To Long Integer(number=w268) -> (32bit integer=w270:i32)
        n85 = call <vilib>:"Mean PtByPt.vi"("x"=w267, "sample length"=w270) -> ("mean"=w269:dbl)  [unwired: 1 in, 2 out]
        n86 = formula code="ScaledOut = ((Vin-Offset)*Slope);\nVout=Vin;"("Vin"=w269, "Slope"=w266, "Offset"=w265) -> ("ScaledOut"=w264:dbl, "Vout"=w263:dbl)
      }
      frame 23 {
        # "24    CH23\t\tPins  31/32\t Fuel Temp (Panel)  TC2"
        # "Ind# USB#2"
        n87 = To Long Integer(number=w276) -> (32bit integer=w278:i32)
        n88 = call <vilib>:"Mean PtByPt.vi"("x"=w275, "sample length"=w278) -> ("mean"=w277:dbl)  [unwired: 1 in, 2 out]
        n89 = formula code="ScaledOut = ((Vin-Offset)*Slope);\nVout=Vin;"("Vin"=w277, "Slope"=w274, "Offset"=w273) -> ("ScaledOut"=w272:dbl, "Vout"=w271:dbl)
      }
      frame 24 {
        # "25    CH24\t\tPins \t47/48\t Lube Res Temp     TC3"
        # "Ind# USB#2"
        n90 = To Long Integer(number=w284) -> (32bit integer=w286:i32)
        n91 = call <vilib>:"Mean PtByPt.vi"("x"=w283, "sample length"=w286) -> ("mean"=w285:dbl)  [unwired: 1 in, 2 out]
        n92 = formula code="ScaledOut = ((Vin-Offset)*Slope);\nVout=Vin;"("Vin"=w285, "Slope"=w282, "Offset"=w281) -> ("ScaledOut"=w280:dbl, "Vout"=w279:dbl)
      }
      frame 25 {
        # "26    CH25\t\tPins  49/50\t Lub  Temp (Panel) TC4"
        # "Ind# USB#2"
        n93 = To Long Integer(number=w292) -> (32bit integer=w294:i32)
        n94 = call <vilib>:"Mean PtByPt.vi"("x"=w291, "sample length"=w294) -> ("mean"=w293:dbl)  [unwired: 1 in, 2 out]
        n95 = formula code="ScaledOut = ((Vin-Offset)*Slope);\nVout=Vin;"("Vin"=w293, "Slope"=w290, "Offset"=w289) -> ("ScaledOut"=w288:dbl, "Vout"=w287:dbl)
      }
      frame 26 {
        # "27    CH26\t\tPins  51/52\t RTD"
        # "Ind# USB#2"
        n96 = To Long Integer(number=w300) -> (32bit integer=w302:i32)
        n97 = call <vilib>:"Mean PtByPt.vi"("x"=w299, "sample length"=w302) -> ("mean"=w301:dbl)  [unwired: 1 in, 2 out]
        n98 = formula code="ScaledOut = ((Vin-Offset)*Slope);\nVout=Vin;"("Vin"=w301, "Slope"=w298, "Offset"=w297) -> ("ScaledOut"=w296:dbl, "Vout"=w295:dbl)
      }
      frame 27 {
        # "28    CH27\t\tPins  53/54\t TM1 Amps"
        # "Ind# USB#2"
        n99 = To Long Integer(number=w308) -> (32bit integer=w310:i32)
        n100 = call <vilib>:"Mean PtByPt.vi"("x"=w307, "sample length"=w310) -> ("mean"=w309:dbl)  [unwired: 1 in, 2 out]
        n101 = formula code="ScaledOut = ((Vin-Offset)*Slope);\nVout=Vin;"("Vin"=w309, "Slope"=w306, "Offset"=w305) -> ("ScaledOut"=w304:dbl, "Vout"=w303:dbl)
      }
      frame 28 {
        # "29    CH28\t\tPins  56/57\t TM2 Volts"
        # "Ind# USB#2"
        n102 = To Long Integer(number=w316) -> (32bit integer=w318:i32)
        n103 = call <vilib>:"Mean PtByPt.vi"("x"=w315, "sample length"=w318) -> ("mean"=w317:dbl)  [unwired: 1 in, 2 out]
        n104 = formula code="ScaledOut = ((Vin-Offset)*Slope);\nVout=Vin;"("Vin"=w317, "Slope"=w314, "Offset"=w313) -> ("ScaledOut"=w312:dbl, "Vout"=w311:dbl)
      }
      frame 29 {
        # "30    CH29\t\tPins  58/59\t TM2 Amps"
        # "Ind# USB#2"
        n105 = To Long Integer(number=w324) -> (32bit integer=w326:i32)
        n106 = call <vilib>:"Mean PtByPt.vi"("x"=w323, "sample length"=w326) -> ("mean"=w325:dbl)  [unwired: 1 in, 2 out]
        n107 = formula code="ScaledOut = ((Vin-Offset)*Slope);\nVout=Vin;"("Vin"=w325, "Slope"=w322, "Offset"=w321) -> ("ScaledOut"=w320:dbl, "Vout"=w319:dbl)
      }
      frame 30 {
        # "31    CH30\t\tPins  61/62  Solenoid Power Volts"
        # "Ind# USB#2"
        n108 = To Long Integer(number=w332) -> (32bit integer=w334:i32)
        n109 = call <vilib>:"Mean PtByPt.vi"("x"=w331, "sample length"=w334) -> ("mean"=w333:dbl)  [unwired: 1 in, 2 out]
        n110 = formula code="ScaledOut = ((Vin-Offset)*Slope);\nVout=Vin;"("Vin"=w333, "Slope"=w330, "Offset"=w329) -> ("ScaledOut"=w328:dbl, "Vout"=w327:dbl)
      }
      frame 31 {
        # "32    CH31\t\tPins  63/64  Solenoid Power Amps"
        # "Ind# USB#2"
        n111 = To Long Integer(number=w340) -> (32bit integer=w342:i32)
        n112 = call <vilib>:"Mean PtByPt.vi"("x"=w339, "sample length"=w342) -> ("mean"=w341:dbl)  [unwired: 1 in, 2 out]
        n113 = formula code="ScaledOut = ((Vin-Offset)*Slope);\nVout=Vin;"("Vin"=w341, "Slope"=w338, "Offset"=w337) -> ("ScaledOut"=w336:dbl, "Vout"=w335:dbl)
      }
    }
  }
  "ScaledOut" <- w10
  n114 = Number To Fractional String(number=w19, precision (6)=i16 6) -> (F-format string=→"Vout":string[])  [unwired: 2 out]
  n115 = Number To Fractional String(number=w10, precision (6)=i16 6) -> (F-format string=→"ScaledOut":string[])  [unwired: 2 out]
  "Allow Zero?" <- "Allow Zero?"
  "Offset Data" <- "Offset Data"
  "error out" <- "error in"
